vi "Colour detection.vi"() -> ()   [LabVIEW 2018]
uses:
  Underlying VI's/Modified webcam FGV/Webcam AE.ctl
  <vilib>/userdefined/High Color/IMAQdx.ctl
panel:
  out "Colour output boolean cluster":T1
  in  "stop":bool
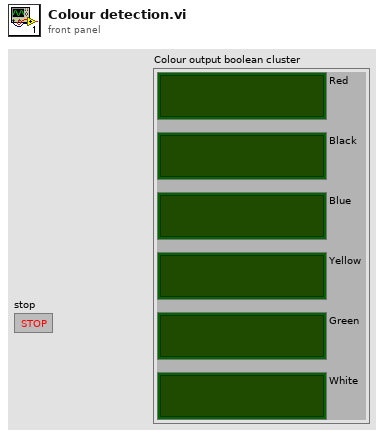
[diagram p1: front panel]
types:
  T1 = cluster{"Red":bool, "Black":bool, "Blue":bool, "Yellow":bool, "Green":bool, "White":bool}
  T2 = typedef "Webcam AE.ctl" = enum16{"Initialize Camera", "Open Camera", "Continuous Acquisition", "Close Camera", "Retrieve Image", "Dispose Camera Image Buffer"}
  T3 = typedef "IMAQdx.ctl" = refnum<k21>
  T4 = typedef "IMAQ Image.ctl" = refnum<image>
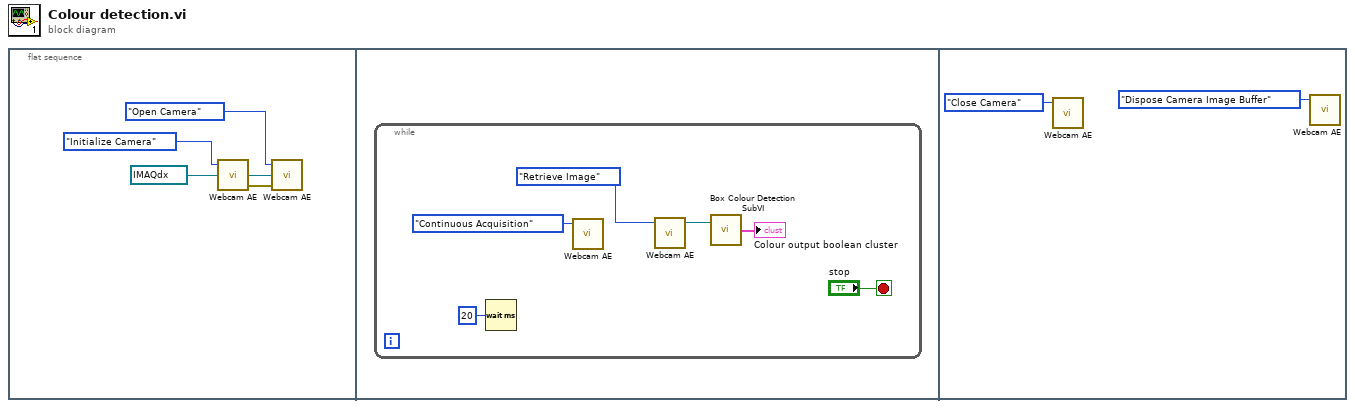
[diagram p0: block diagram]
diagram:
  n1 = flat-sequence {
    frame #0 {
      n2 = call "Webcam AE.vi"("Session In"=T3 "cam1", "Camera states"=Webcam_AE."Initialize Camera") -> ("error out"=w4:errorcluster, "Session Out"=w5:T3)  [unwired: 1 in, 1 out]
      n3 = call "Webcam AE.vi"("error in (no error)"=w4, "Session In"=w5, "Camera states"=Webcam_AE."Open Camera") -> ()  [unwired: 3 out]
    }
    frame #1 {
      n4 = while {
        stop <- "stop" stop-if-true
        n5 = Wait (ms)(milliseconds to wait=u32 20) -> ()  [unwired: 1 out]
        n6 = call "Webcam AE.vi"("Camera states"=Webcam_AE."Continuous Acquisition") -> ()  [unwired: 2 in, 3 out]
        n7 = call "Webcam AE.vi"("Camera states"=Webcam_AE."Retrieve Image") -> ("Image Out"=w7:T4)  [unwired: 2 in, 2 out]
        n8 = call "Box Colour Detection SubVI.vi"("Image In"=w7) -> ("Colour output boolean cluster"=→"Colour output boolean cluster":T1)  [unwired: 1 in, 2 out]
      }
    }
    frame #2 {
      n9 = call "Webcam AE.vi"("Camera states"=Webcam_AE."Close Camera") -> ()  [unwired: 2 in, 3 out]
      n10 = call "Webcam AE.vi"("Camera states"=Webcam_AE."Dispose Camera Image Buffer") -> ()  [unwired: 2 in, 3 out]
    }
  }
